vi "TP3.vi"() -> ()   [LabVIEW 2017]
panel:
  in  "Minute":dbl
  in  "Heure":dbl
  out "HORLOGE":string
  in  "?":bool
  in  "stop":bool
  out "Alarm LED":bool
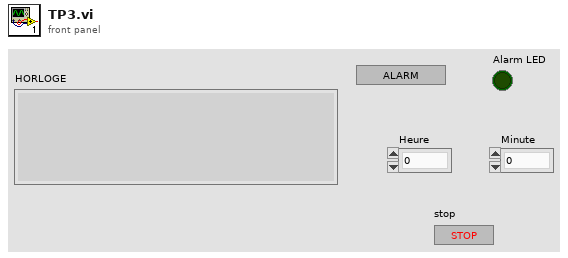
[diagram p1: front panel]
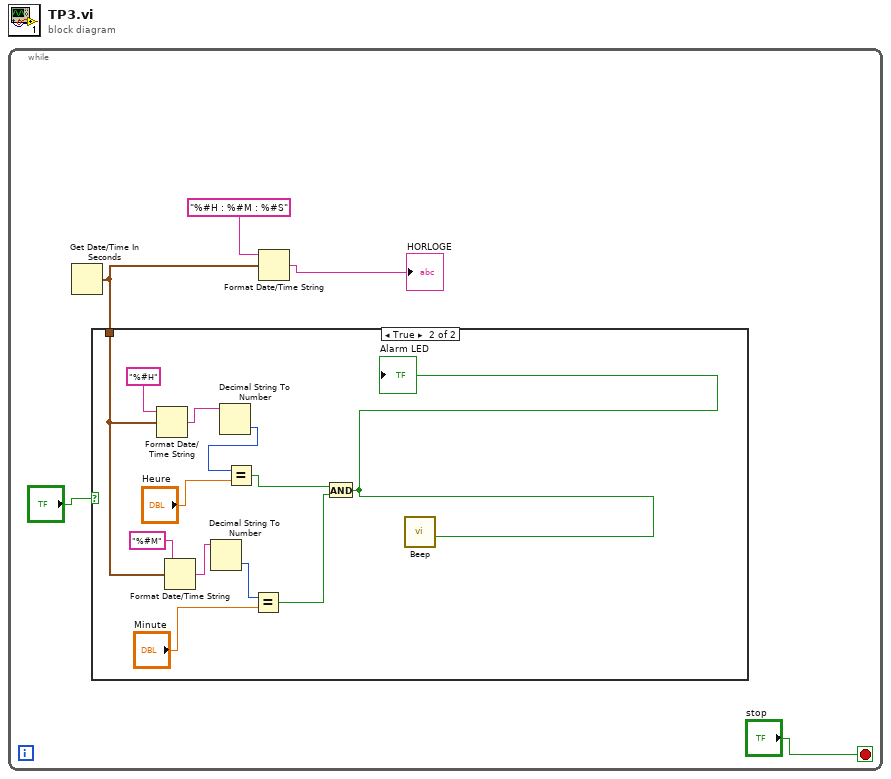
[diagram p0: block diagram]
diagram:
  n1 = while {
    stop <- "stop" stop-if-true
    n2 = Get Date/Time In Seconds() -> (seconds since 1Jan1904=w2:timestamp)
    n3 = case shown="True" "?" {
      tunnel: w2 -> [_ w7]
      frame False {
      }
      frame True {
        n4 = Format Date/Time String(time format string (%c)="%#H", seconds (now)=w7) -> (date/time string=w15:string)  [unwired: 1 in]
        n5 = Format Date/Time String(time format string (%c)="%#M", seconds (now)=w7) -> (date/time string=w11:string)  [unwired: 1 in]
        n6 = Decimal String To Number(string=w11) -> (number=w10:i32)  [unwired: 2 in, 1 out]
        n7 = Decimal String To Number(string=w15) -> (number=w14:i32)  [unwired: 2 in, 1 out]
        n8 = Equal?(x=w14, y="Heure") -> (x = y?=w8:bool)
        n9 = Equal?(x=w10, y="Minute") -> (x = y?=w9:bool)
        n10 = And(x=w8, y=w9) -> (x .and. y?=w6:bool)
        "Alarm LED" <- w6
        n11 = call <vilib>:"Beep.vi"("use system alert? (T)"=w6) -> ()  [unwired: 11 in]
      }
    }
    n12 = Format Date/Time String(time format string (%c)="%#H : %#M : %#S", seconds (now)=w2) -> (date/time string=→"HORLOGE":string)  [unwired: 1 in]
  }
